vi "numeric_function.vi"() -> ()   [LabVIEW 2019]
uses:
  <vilib>/numeric/Random Number (Range) DBL.vi
panel:
  out "x*2^n":dbl
  out "number":dbl
  in  "z":dbl
  out "-1, 0, 1":dbl
  out "1/x":dbl
  out "-x":dbl
  out "sqrt(x)":dbl
  out "x-1":dbl
  out "x+1":dbl
  out "floor(x/y)":dbl
  out "x-y*floor(x/y)":dbl
  out "x/y":dbl
  out "x*y":dbl
  out "x-y":dbl
  out "x+y":dbl
  in  "y":dbl
  in  "x":dbl
  # "adddition"
  # "remainder"
  # "subtraction"
  # "quotient"
  # "multiplication"
  # "division"
  # "increment"
  # "decrement"
  # "square root"
  # "negate"
  # "reciprocal"
  # "sign"
  # "scale  by power 2"
  # "random number"
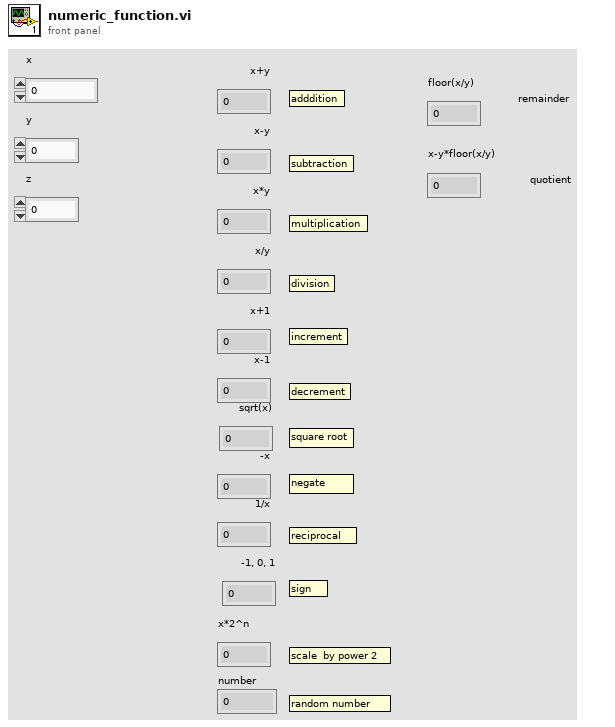
[diagram p1: front panel]
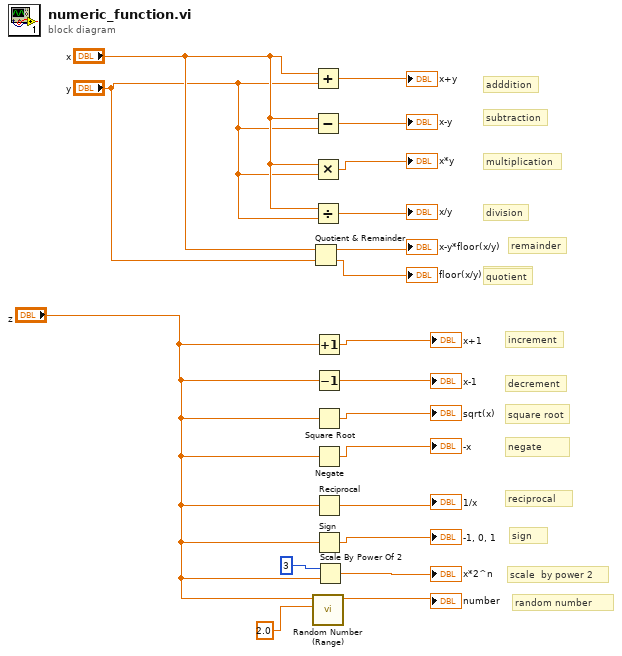
[diagram p0: block diagram]
diagram:
  # "remainder"
  # "random number"
  # "scale  by power 2"
  # "sign"
  # "reciprocal"
  # "negate"
  # "square root"
  # "decrement"
  # "increment"
  # "quotient"
  # "quotient"
  # "division"
  # "multiplication"
  # "subtraction"
  # "adddition"
  n1 = Quotient & Remainder(x="x", y="y") -> (x-y*floor(x/y)=→"x-y*floor(x/y)":dbl, floor(x/y)=→"floor(x/y)":dbl)
  n2 = Add(x="x", y="y") -> (x+y=→"x+y":dbl)
  n3 = Subtract(x="x", y="y") -> (x-y=→"x-y":dbl)
  n4 = Multiply(x="x", y="y") -> (x*y=→"x*y":dbl)
  n5 = Divide(x="x", y="y") -> (x/y=→"x/y":dbl)
  n6 = call-poly <vilib>:"Random Number (Range).vi"("lower bound (0)"=2.0, "upper bound (100)"="z") -> ("number"=→"number":dbl)  [unwired: 9 in]
  n7 = Increment(x="z") -> (x+1=→"x+1":dbl)
  n8 = Decrement(x="z") -> (x-1=→"x-1":dbl)
  n9 = Square Root(x="z") -> (sqrt(x)=→"sqrt(x)":dbl)
  n10 = Negate(x="z") -> (-x=→"-x":dbl)
  n11 = Reciprocal(x="z") -> (1/x=→"1/x":dbl)
  n12 = Sign(1:"z") -> (0:→"-1, 0, 1":dbl)
  n13 = Scale By Power Of 2(n=i16 3, x="z") -> (x*2^n=→"x*2^n":dbl)
